vi "Create and Return Class DVR Refnum.vi"(8 "error in (no error)":errorcluster, 10 "Path to Save DVR Class Control":path, 11 "Class Path":path) -> (0 "error out":errorcluster, 3 "DVR Class Control Path Out":path)   [LabVIEW 2016, in "SLL Class DVR API Generator.lvlib"]
uses:
  SLL Class DVR API Generator.lvlib
  <vilib>/Utility/traverseref.llb/TRef TravTarget.ctl
  <vilib>/Utility/traverseref.llb/VI Scripting - Traverse.lvlib
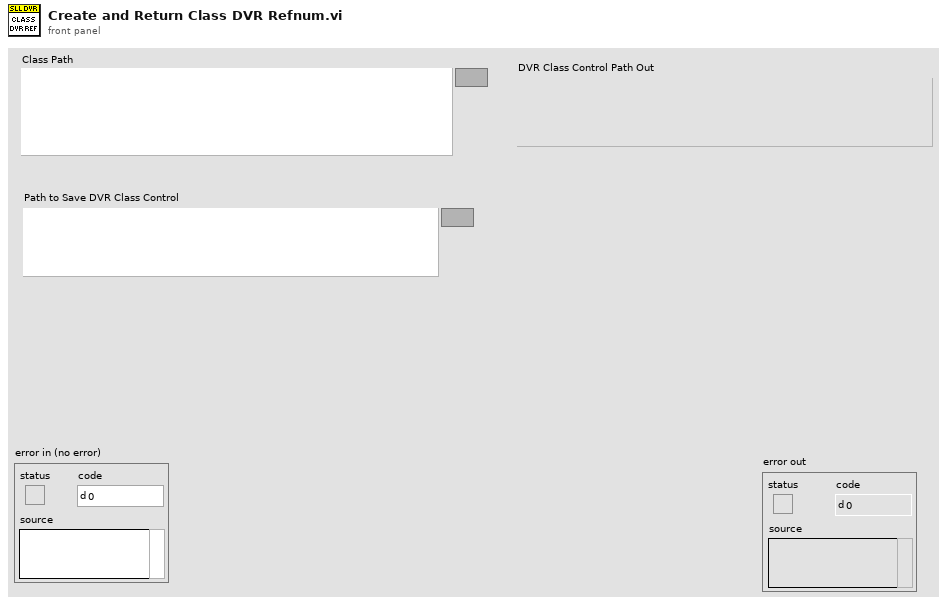
[diagram p1: front panel]
types:
  T1 = enum8{"Probe", "Diagram", "Panel Control", "3D Panel Control", "Dialog Panel Control", "Panel Indicator", "3D Panel Indicator", "Dialog Panel Indicator", "Power PC Control", "Power PC Indicator", "Silver Control", "Silver Indicator"}
  T2 = enum32{"invalid VI type", "Standard VI", "Control VI", "Global VI", "Polymorphic VI", "Configuration VI", "SubSystem", "Facade VI", "Method VI", "Statechart Diagram VI"}
  T3 = typedef "TRef TravTarget.ctl" = enum16{"FP", "BD", "Other"}
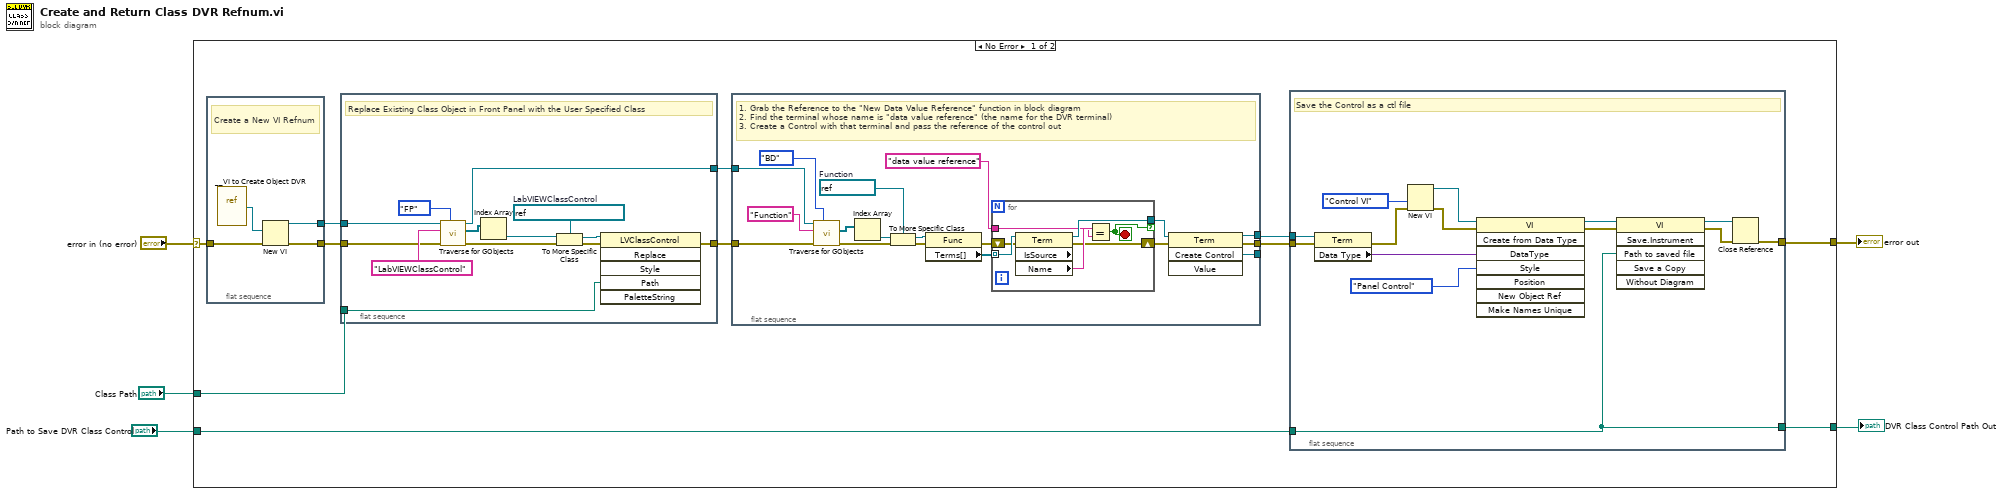
[diagram p0: block diagram]
diagram:
  n1 = case shown="No Error" "error in (no error)" {
    selector: "error in (no error)" -> [w12 w74]
    tunnel: [w7 w74] -> w5
    tunnel: "Class Path" -> [w11 _]
    tunnel: "Path to Save DVR Class Control" -> [w8 w73]
    tunnel: [w6 w73] -> w1
    frame No Error {
      n2 = flat-sequence {
        tunnel: [w71] -> w14
        tunnel: [w70] -> w13
        tunnel: w12 -> [w69]
        frame #0 {
          # "Create a New VI Refnum"
          n3 = vi-ref "__VI to Create Object DVR.vi"() -> (w72:refnum<vi>)
          n4 = New VI(8:w69, 10:w72) -> (0:w70:errorcluster, 3:w71:refnum<vi>)  [unwired: 5 in]
        }
      }
      n5 = flat-sequence {
        tunnel: [w60] -> w16
        tunnel: [w59] -> w15
        tunnel: w14 -> [w58]
        tunnel: w13 -> [w57]
        tunnel: w11 -> [w56]
        frame #0 {
          w66 = refnum<vi> refnum  # LabVIEWClassControl
          # "Replace Existing Class Object in Front Panel with the User Specified Class"
          n6 = call <vilib>:"Traverse for GObjects.vi"("Traverse Target"=TRef_TravTarget."FP", "error in (no error)"=w57, "Class Name"="LabVIEWClassControl", "VI Refnum"=w58) -> ("error out"=w62:errorcluster, "References"=w64:refnum<vi>[], "dup VI Refnum"=w59:refnum<vi>)  [unwired: 4 in, 1 out]
          n7 = Index Array(array=w64) -> (element=w63:refnum<vi>)  [unwired: 1 in]
          n8 = To More Specific Class(target class=w66, reference=w63, error in=w62) -> (specific class reference=w65:refnum<vi>, error out=w61:errorcluster)
          n9 = invoke class="LVClassControl" method="Replace"(reference=w65, error in=w61, "Path"=w56) -> (error out=w60:errorcluster)  [unwired: 3 in, 5 out]
        }
      }
      n10 = flat-sequence {
        tunnel: w16 -> [w48]
        tunnel: w15 -> [w45]
        tunnel: [w37] -> _
        tunnel: [w32] -> w10
        tunnel: [w31] -> w9
        frame #0 {
          w42 = refnum<vi> refnum  # Function
          # "1. Grab the Reference to the \"New Data Value Reference\" function in block diagram\n2. Find the terminal whose name is \"data value reference\" (the name for the DVR terminal)\n3. Create a Control with that terminal and pass the reference of the control out"
          n11 = call <vilib>:"Traverse for GObjects.vi"("Traverse Target"=TRef_TravTarget."BD", "error in (no error)"=w48, "Class Name"="Function", "VI Refnum"=w45) -> ("error out"=w36:errorcluster, "References"=w44:refnum<vi>[])  [unwired: 4 in, 2 out]
          n12 = Index Array(array=w44) -> (element=w43:refnum<vi>)  [unwired: 1 in]
          n13 = To More Specific Class(target class=w42, reference=w43, error in=w36) -> (specific class reference=w41:refnum<vi>, error out=w35:errorcluster)
          n14 = property class="Func"(reference=w41, error in=w35) -> (error out=w34:errorcluster, "Terms[]"=w40:refnum<vi>[])  [unwired: 1 out]
          n15 = for {
            tunnel: w40 -> [w55] mode=indexing
            tunnel: [w54] -> w39 if=w51
            tunnel: "data value reference" -> [w52]
            shift-right: [w49] -> w33
            shift-left: w34 -> [w50]
            stop <- w51 stop-if-true
            n16 = property class="Term" props=["IsSource", "Name"](reference=w55, error in=w50) -> (reference out=w54:refnum<vi>, error out=w49:errorcluster, "Name"=w53:string)  [unwired: 1 out]
            n17 = Equal?(x=w53, y=w52) -> (x = y?=w51:bool)
          }
          n18 = invoke class="Term" method="Create Control"(reference=w39, error in=w33) -> (reference out=w31:refnum<vi>, error out=w32:errorcluster, "Create Control"=w37:refnum<vi>)  [unwired: 2 in, 1 out]
        }
      }
      n19 = flat-sequence {
        tunnel: w9 -> [w20]
        tunnel: [w19] -> w7
        tunnel: w10 -> [w18]
        tunnel: w8 -> [w17]
        tunnel: [w17] -> w6
        frame #0 {
          # "Save the Control as a ctl file"
          n20 = property class="Term"(reference=w20, error in=w18) -> (error out=w30:errorcluster, "Data Type"=w23:variant)  [unwired: 1 out]
          n21 = New VI(8:w30, 9:T2."Control VI" ("vi type (standard vi)")) -> (0:w28:errorcluster, 3:w22:refnum<vi>)  [unwired: 5 in]
          n22 = invoke class="VI" method="Create from Data Type"(reference=w22, error in=w28, "DataType"=w23, "Style"=T1."Panel Control") -> (reference out=w25:refnum<vi>, error out=w29:errorcluster)  [unwired: 4 in, 6 out]
          n23 = invoke class="VI" method="Save.Instrument"(reference=w25, error in=w29, "Path to saved file"=w17) -> (reference out=w26:refnum<vi>, error out=w27:errorcluster)  [unwired: 3 in, 4 out]
          n24 = Close Reference(reference=w26, error in (no error)=w27) -> (error out=w19:errorcluster)
        }
      }
    }
    frame Error {
    }
  }
  "error out" <- w5
  "DVR Class Control Path Out" <- w1
